vi "Init Msg Output.vi"() -> (2 "Msg Output":refnum<class "Msg Output.lvclass">)   [LabVIEW 2020, in "jettl.lvlib" / "Stopping jettl Msg.lvlib" / "Stopping Msg Output.lvlib"]
doc: "jettl 6.12.1.94\nNathan Davis - Nathan Davis\nCopyright (c) 2026, Nathan Davis\nMIT"
uses:
  Stopping Msg Output.lvlib
  Msg Output/Msg Output.lvclass
  Stopping Msg Output/Stopping Msg Output.lvclass
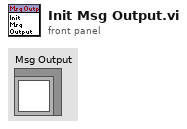
[diagram p1: front panel]
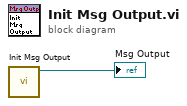
[diagram p0: block diagram]
diagram:
  n1 = call "Init Msg Output.vi"() -> ("Stopping Msg Output out"=→"Msg Output":refnum<class "Stopping Msg Output.lvclass">)  [unwired: 11 in]
